vi "采配水启动流程.vi"() -> ()   [LabVIEW 2016]
uses:
  <vilib>/Utility/miscctls.llb/LVPointTypeDef.ctl
panel:
  in  "步骤时间/秒":T1={"步骤1时间"=2, "步骤2时间"=4, "步骤3时间"=2, "步骤4时间"=5, "步骤5时间"=6, "步骤6时间"=3, "步骤7时间"=2400, "步骤8时间"=7, "步骤9时间"=8, "步骤10时间"=6}
  out "启动记录":string
  out "流程运行中":bool
  out "启动次数":i32
  out "日期/时间":string
  out "运行状态":string
  out "步骤运行时间/秒":i32
  out "流程结束":bool
  out "当前步骤":T2(ring)
  # "采配水模块"
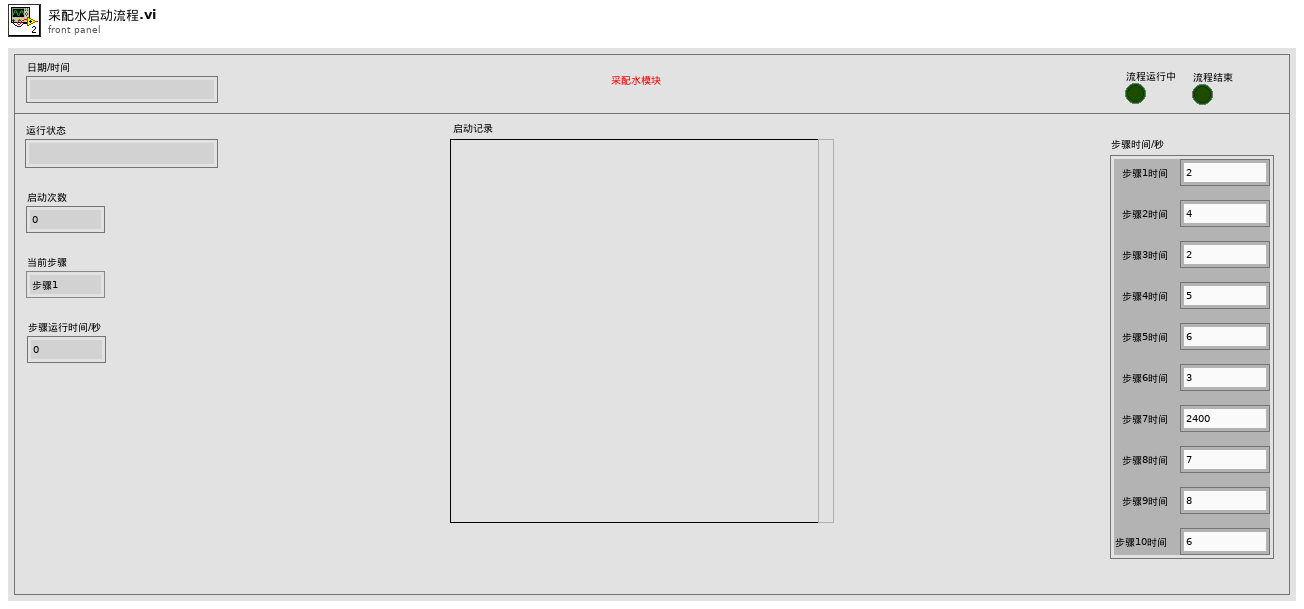
[diagram p1: front panel]
types:
  T1 = cluster{"步骤1时间":i32, "步骤2时间":i32, "步骤3时间":i32, "步骤4时间":i32, "步骤5时间":i32, "步骤6时间":i32, "步骤7时间":i32, "步骤8时间":i32, "步骤9时间":i32, "步骤10时间":i32}
  T2 = enum16{"步骤1", "步骤2", "步骤3", "步骤4", "步骤5", "步骤6", "步骤7", "步骤8", "步骤9", "步骤10"}
  T3 = enum16{"write register", "read register", "write and read register", "write coil", "read coil"}
  T4 = typedef "LVPointTypeDef.ctl" = cluster{"Horizontal":i16, "Vertical":i16}
  T5 = cluster{"R0":i16, "R1":i16, "R2":i16, "R3":i16, "R4":i16, "R5":i16, "R6":i16, "R7":i16, "R8":i16, "R9":i16, "R10":i16, "R11":i16, "R12":i16, "R13":i16, "R14":i16, "R15":i16, "R16":i16, "R17":i16, "R18":i16, "R19":i16, "R20":i16, "R21":i16, "R22":i16, "R23":i16, "R24":i16, "R25":i16}
  T6 = enum32{"Bad", "Idle", "Run top level", "Running"}
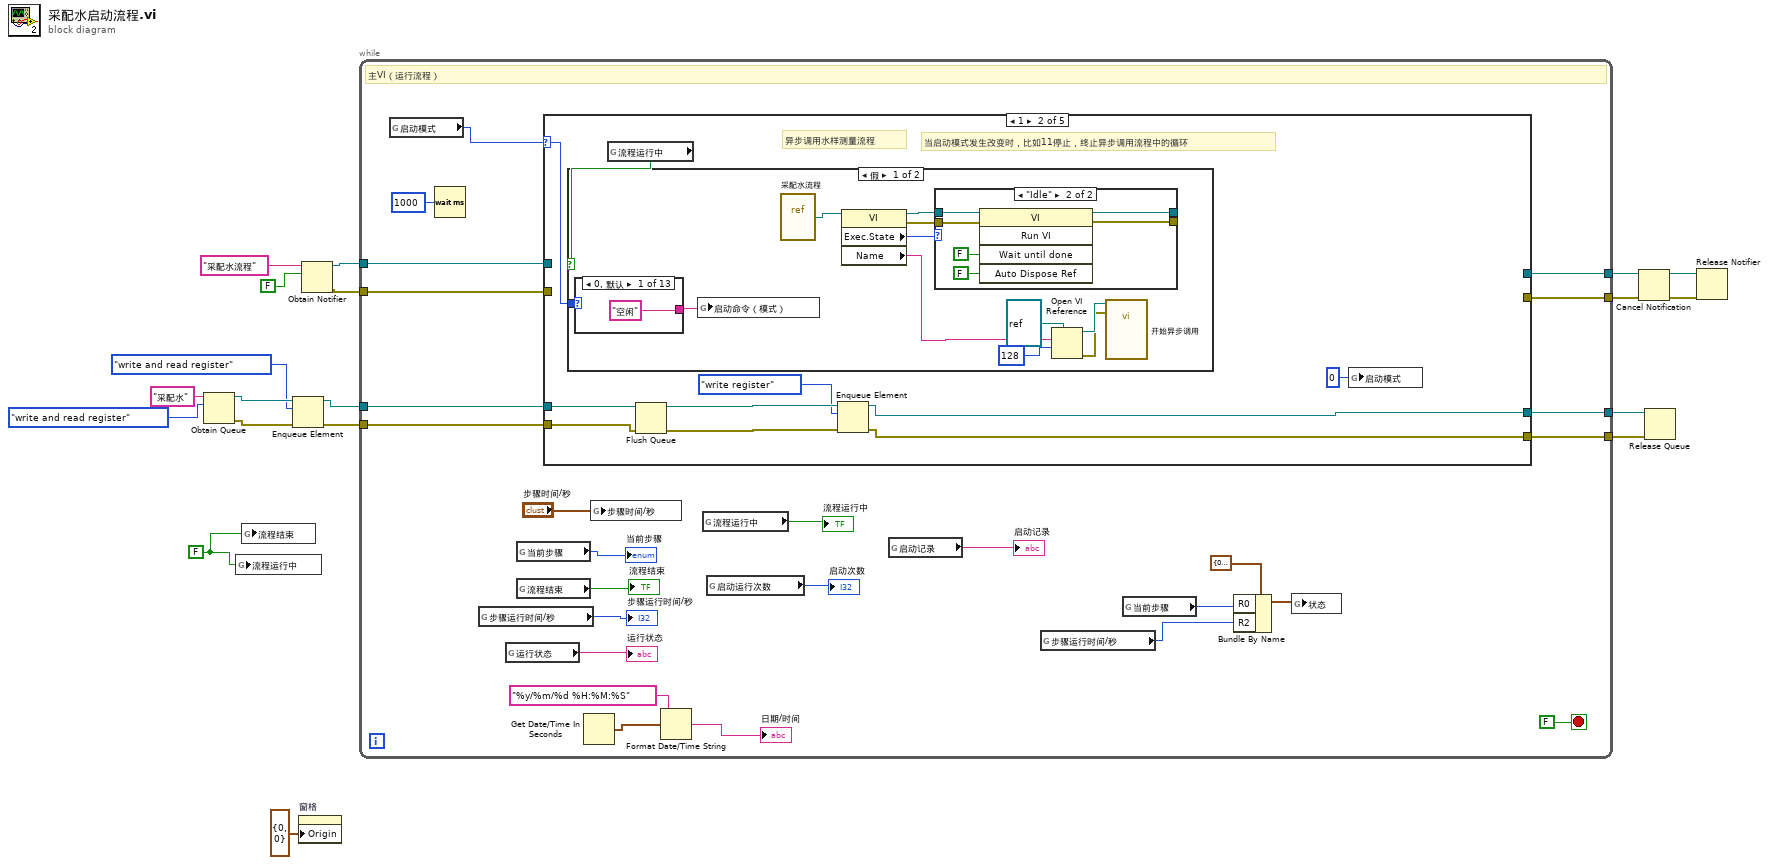
[diagram p0: block diagram]
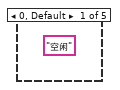
[diagram p2: hidden frame]
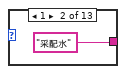
[diagram p4: hidden frame]
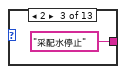
[diagram p5: hidden frame]
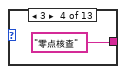
[diagram p6: hidden frame]
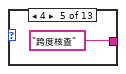
[diagram p7: hidden frame]
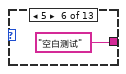
[diagram p8: hidden frame]
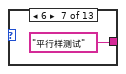
[diagram p9: hidden frame]
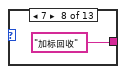
[diagram p10: hidden frame]
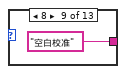
[diagram p11: hidden frame]
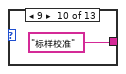
[diagram p12: hidden frame]
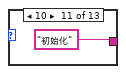
[diagram p13: hidden frame]
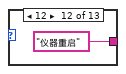
[diagram p14: hidden frame]
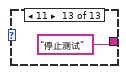
[diagram p15: hidden frame]
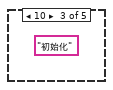
[diagram p17: hidden frame]
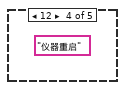
[diagram p18: hidden frame]
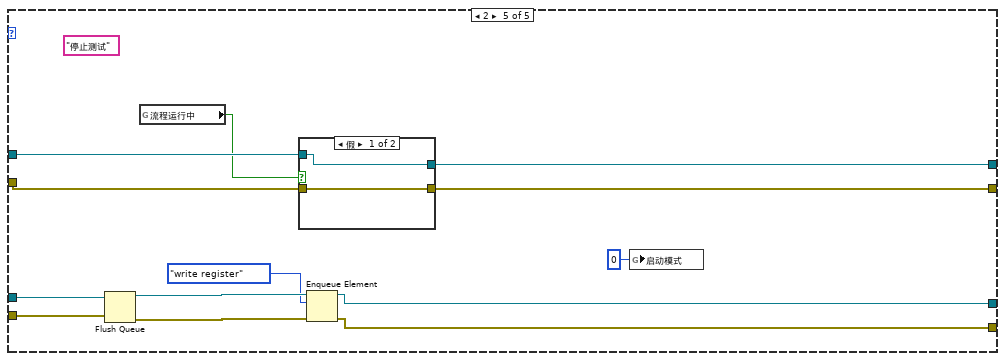
[diagram p19: hidden frame]
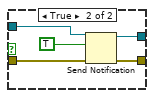
[diagram p20: hidden frame]
diagram:
  w10 = FALSE ("流程结束")
  n1 = Obtain Queue(name (unnamed)="采配水" ("名称（未命名）"), element data type=T3."write and read register") -> (queue out=w7:refnum<queue>, error out=w6:errorcluster)  [unwired: 3 in, 1 out]
  n2 = global write "采配水全局.vi" "流程运行中"(w10) -> ()
  n3 = global write "采配水全局.vi" "流程结束"(w10) -> ()
  n4 = Enqueue Element(queue=w7, element=T3."write and read register", error in (no error)=w6) -> (queue out=w4:refnum<queue>, error out=w3:errorcluster)  [unwired: 1 in, 1 out]
  n5 = property on="窗格" class="Pane"("Origin"=T4 {"Horizontal"=0, "Vertical"=0} ("原点")) -> ()  [unwired: 2 in, 2 out]
  n6 = Obtain Notifier(name (unnamed)="采配水流程" ("名称（未命名）"), notification data type=FALSE) -> (notifier out=w15:refnum<notifier>, error out=w14:errorcluster)  [unwired: 2 in, 1 out]
  n7 = while {
    tunnel: w14 -> [w43]
    tunnel: w15 -> [w42]
    tunnel: [w41] -> w18
    tunnel: [w40] -> w19
    tunnel: w4 -> [w25]
    tunnel: w3 -> [w24]
    tunnel: [w23] -> w2
    tunnel: [w22] -> w1
    stop <- FALSE stop-if-true
    # "主VI（运行流程）"
    n8 = global read "采配水全局.vi" "启动模式"() -> (w20:u16)
    n9 = Wait (ms)(milliseconds to wait=u32 1000 ("等待时间（毫秒）")) -> ()  [unwired: 1 out]
    n10 = global read "采配水全局.vi" "步骤运行时间/秒"() -> (→"步骤运行时间/秒":i32)
    n11 = global read "采配水全局.vi" "运行状态"() -> (→"运行状态":string)
    n12 = global read "采配水全局.vi" "当前步骤"() -> (→"当前步骤":T2)
    n13 = global read "采配水全局.vi" "流程结束"() -> (→"流程结束":bool)
    n14 = case shown="1" w20 {
      selector: w20 -> [_ w55 _ _ _]
      tunnel: w43 -> [_ _ _ _ w100]
      tunnel: w42 -> [_ _ _ _ w99]
      tunnel: [_ _ _ _ w98] -> w41
      tunnel: [_ _ _ _ w97] -> w40
      tunnel: w25 -> [_ w51 _ _ w93]
      tunnel: w24 -> [_ w50 _ _ w92]
      tunnel: [_ w49 _ _ w91] -> w23
      tunnel: [_ w48 _ _ w90] -> w22
      frame 0, Default {
        (unwired) "空闲"
      }
      frame 1 {
        # "当启动模式发生改变时，比如11停止，终止异步调用流程中的循环"
        # "异步调用水样测量流程"
        n15 = global read "采配水全局.vi" "流程运行中"() -> (w47:bool)
        n16 = case shown="假" w47 {
          tunnel: w55 -> [w57 _]
          frame False {
            n17 = case shown="0, 默认" w57 {
              tunnel: ["空闲" "采配水" "采配水停止" "零点核查" "跨度核查" "空白测试" "平行样测试" "加标回收" "空白校准" "标样校准" "初始化" "仪器重启" "停止测试"] -> w56
              frame 0, Default {
              }
              frame 1 {
              }
              frame 2 {
              }
              frame 3 {
              }
              frame 4 {
              }
              frame 5 {
              }
              frame 6 {
              }
              frame 7 {
              }
              frame 8 {
              }
              frame 9 {
              }
              frame 10 {
              }
              frame 12 {
              }
              frame 11 {
              }
            }
            n18 = global write "采配水全局.vi" "启动命令（模式）"(w56) -> ()
            n19 = vi-ref "采配水流程.vi"() -> (w66:refnum<vi>)
            n20 = property class="VI"(reference=w66) -> (reference out=w65:refnum<vi>, error out=w63:errorcluster, "Exec.State"=w64:T6, "Name"=w58:string)  [unwired: 1 in]
            n21 = case shown="\"Idle\"" w64 {
              tunnel: w65 -> [w68 w74]
              tunnel: [w68 w73] -> _
              tunnel: w63 -> [w67 w70]
              tunnel: [w67 w69] -> _
              frame "Bad", Default {
              }
              frame "Idle" {
                n22 = invoke class="VI" method="Run VI"(reference=w74, error in=w70, "Wait until done"=FALSE ("结束前等待"), "Auto Dispose Ref"=FALSE ("自动销毁引用")) -> (reference out=w73:refnum<vi>, error out=w69:errorcluster)  [unwired: 1 in, 3 out]
              }
            }
            n23 = Open VI Reference(type specifier VI Refnum (for type only)=refnum<vi> refnum ("类型说明符VI引用句柄（仅用于类型）"), vi path=w58, options=128 ("选项")) -> (vi reference=w62:refnum<vi>, error out=w60:errorcluster)  [unwired: 3 in]
            n24 = call-by-ref "开始异步调用"(reference=w62, error in=w60) -> ()  [unwired: 12 in, 2 out]
          }
          frame True {
          }
        }
        n25 = Flush Queue(queue=w51, error in (no error)=w50) -> (queue out=w54:refnum<queue>, error out=w53:errorcluster)  [unwired: 1 out]
        n26 = Enqueue Element(queue=w54, element=T3."write register", error in (no error)=w53) -> (queue out=w49:refnum<queue>, error out=w48:errorcluster)  [unwired: 1 in, 1 out]
        n27 = global write "采配水全局.vi" "启动模式"(u16 0 ("启动模式")) -> ()
      }
      frame 10 {
        (unwired) "初始化"
      }
      frame 12 {
        (unwired) "仪器重启"
      }
      frame 2 {
        (unwired) "停止测试"
        n28 = Flush Queue(queue=w93, error in (no error)=w92) -> (queue out=w96:refnum<queue>, error out=w95:errorcluster)  [unwired: 1 out]
        n29 = global read "采配水全局.vi" "流程运行中"() -> (w89:bool)
        n30 = case shown="假" w89 {
          tunnel: w100 -> [w101 w106]
          tunnel: w99 -> [w102 w105]
          tunnel: [w102 w104] -> w98
          tunnel: [w101 w103] -> w97
          frame False {
          }
          frame True {
            n31 = Send Notification(notification=TRUE ("通知"), notifier=w105, error in (no error)=w106) -> (notifier out=w104:refnum<notifier>, error out=w103:errorcluster)
          }
        }
        n32 = Enqueue Element(queue=w96, element=T3."write register", error in (no error)=w95) -> (queue out=w91:refnum<queue>, error out=w90:errorcluster)  [unwired: 1 in, 1 out]
        n33 = global write "采配水全局.vi" "启动模式"(u16 0 ("启动模式")) -> ()
      }
    }
    n34 = Get Date/Time In Seconds() -> (seconds since 1Jan1904=w39:timestamp)
    n35 = global write "采配水全局.vi" "步骤时间/秒"("步骤时间/秒") -> ()
    n36 = Format Date/Time String(time format string (%c)="%y/%m/%d %H:%M:%S" ("时间格式字符串(%c)"), seconds (now)=w39) -> (date/time string=→"日期/时间":string)  [unwired: 1 in]
    n37 = global read "采配水全局.vi" "流程运行中"() -> (→"流程运行中":bool)
    n38 = global read "采配水全局.vi" "启动运行次数"() -> (→"启动次数":i32)
    n39 = global read "采配水全局.vi" "启动记录"() -> (→"启动记录":string)
    n40 = global read "采配水全局.vi" "步骤运行时间/秒"() -> (w26:i32)
    n41 = global read "采配水全局.vi" "当前步骤"() -> (w27:T2)
    n42 = Bundle By Name(cluster=T5 {"R0"=0, "R1"=0, "R2"=0, "R3"=0, "R4"=0, "R5"=0, "R6"=0, "R7"=0, "R8"=0, "R9"=0, "R10"=0, "R11"=0, "R12"=0, "R13"=0, "R14"=0, "R15"=0, "R16"=0, "R17"=0, "R18"=0, "R19"=0, "R20"=0, "R21"=0, "R22"=0, "R23"=0, "R24"=0, "R25"=0} ("状态"), "R0"=w27, "R2"=w26) -> (w28:T5)
    n43 = global write "采配水全局.vi" "状态"(w28) -> ()
  }
  n44 = Cancel Notification(0:w18, 3:w19) -> (8:w17:refnum<notifier>, 11:w16:errorcluster)  [unwired: 1 out]
  n45 = Release Queue(queue=w2, error in (no error)=w1) -> ()  [unwired: 1 in, 3 out]
  n46 = Release Notifier(notifier=w17, error in (no error)=w16) -> ()  [unwired: 1 in, 3 out]
